vi "Post-Reanimate Hook.vi"(8 "Error In":errorcluster) -> (0 "Error Out":errorcluster)   [LabVIEW 2018, in "Tests.lvlib" / "Toolkit.lvlib" / "Integration.lvlib"]
uses:
  Integration.lvlib
  Hooks/Post-Reanimate.vi
  Support/Reanimate Target.vi
  <vilib>/addons/_JKI Toolkits/Caraya/classes/Test/Test.lvclass
  Tests.lvlib
  <vilib>/addons/_JKI Toolkits/Caraya/classes/Assert/Assert.lvclass
  src/Toolkit/Toolkit.lvlib
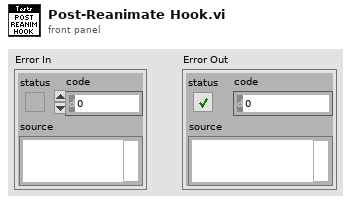
[diagram p1: front panel]
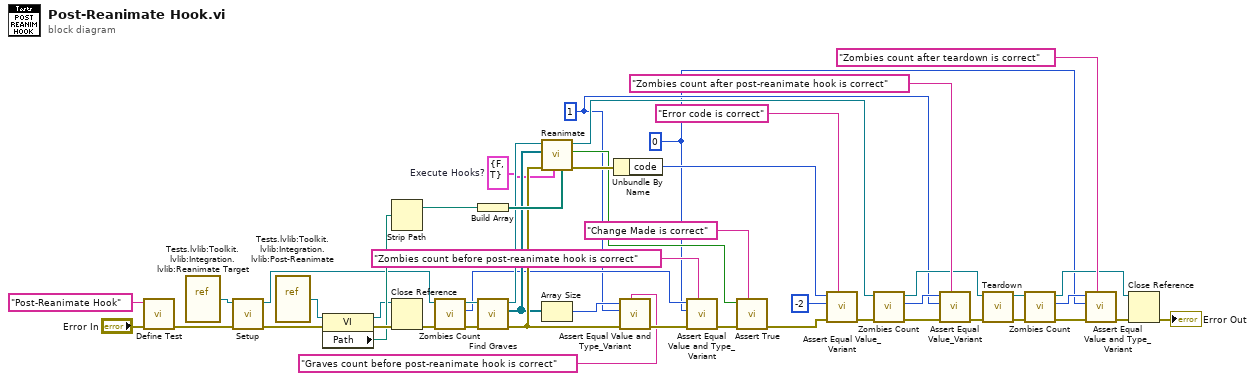
[diagram p0: block diagram]
diagram:
  w2 = 1 ("size(s)")
  w16 = cluster{"Pre":bool, "Post":bool} {"Pre"=FALSE, "Post"=TRUE}  # Execute Hooks?
  w1 = 0 ("size(s)")
  n1 = call <vilib>:"Define Test.vi"("error in (no error)"="Error In", "Label (VI Title)"="Post-Reanimate Hook") -> ("error out"=w44:errorcluster)  [unwired: 9 in]
  n2 = vi-ref "Tests.lvlib:Toolkit.lvlib:Integration.lvlib:Reanimate Target.vi"() -> (w11:refnum<vi>)
  n3 = call "Setup.vi"("Error In"=w44, "VI In"=w11) -> ("Error Out"=w36:errorcluster, "VI Out"=w28:refnum<vi>)  [unwired: 8 in]
  n4 = vi-ref "Tests.lvlib:Toolkit.lvlib:Integration.lvlib:Post-Reanimate.vi"() -> (w12:refnum<vi>)
  n5 = property class="VI"(reference=w12, error in=w36) -> (reference out=w32:refnum<vi>, error out=w35:errorcluster, "Path"=w34:path)
  n6 = Strip Path(path=w34) -> (stripped path=w33:path)  [unwired: 1 out]
  n7 = Close Reference(reference=w32, error in (no error)=w35) -> (error out=w9:errorcluster)
  n8 = call "Zombies Count.vi"("Error In"=w9, "Test Target In"=w28) -> ("Error Out"=w8:errorcluster, "Zombies Count"=w3:i32, "Test Target Out"=w10:refnum<vi>)  [unwired: 7 in]
  n9 = Build Array(w33) -> (w29:path[])
  n10 = call "Find Graves.vi"("Error In"=w8, "VI In"=w10) -> ("Error Out"=w26:errorcluster, "Graves"=w25:refnum<vi>[], "VI Out"=w27:refnum<vi>)  [unwired: 7 in]
  n11 = call "Reanimate.vi"("Hook Search Path"=w29, "Execute Hooks?"=w16, "Error In"=w26, "Graves"=w25, "VI In"=w27) -> ("Error Out"=w23:errorcluster, "Change Made?"=w14:bool, "VI Out"=w18:refnum<vi>)  [unwired: 4 in]
  n12 = Array Size(array=w25) -> (size(s)=w24:i32)
  n13 = Unbundle By Name(w23) -> ("code"=w31:i32)
  n14 = call <vilib>:"Assert Equal Value and Type_Variant.vi"("Label"="Graves count before post-reanimate hook is correct", "error in (no error)"=w26, "Y"=w2, "X"=w24) -> ("error out"=w7:errorcluster)  [unwired: 7 in]
  n15 = call <vilib>:"Assert Equal Value and Type_Variant.vi"("Label"="Zombies count before post-reanimate hook is correct", "error in (no error)"=w7, "Y"=w1, "X"=w3) -> ("error out"=w6:errorcluster)  [unwired: 7 in]
  n16 = call <vilib>:"Assert True.vi"("Label"="Change Made is correct", "error in (no error)"=w6, "True?"=w14) -> ("error out"=w15:errorcluster)  [unwired: 8 in]
  n17 = call <vilib>:"Assert Equal Value_Variant.vi"("Label"="Error code is correct", "error in (no error)"=w15, "Y"=-2 ("code"), "X"=w31) -> ("error out"=w22:errorcluster)  [unwired: 7 in]
  n18 = call "Zombies Count.vi"("Error In"=w22, "Test Target In"=w18) -> ("Error Out"=w21:errorcluster, "Zombies Count"=w20:i32, "Test Target Out"=w19:refnum<vi>)  [unwired: 7 in]
  n19 = call <vilib>:"Assert Equal Value_Variant.vi"("Label"="Zombies count after post-reanimate hook is correct", "error in (no error)"=w21, "Y"=w2, "X"=w20) -> ("error out"=w17:errorcluster)  [unwired: 7 in]
  n20 = call "Teardown.vi"("Error In"=w17, "VI In"=w19) -> ("Error Out"=w39:errorcluster, "VI Out"=w41:refnum<vi>)  [unwired: 8 in]
  n21 = call "Zombies Count.vi"("Error In"=w39, "Test Target In"=w41) -> ("Error Out"=w38:errorcluster, "Zombies Count"=w37:i32, "Test Target Out"=w40:refnum<vi>)  [unwired: 7 in]
  n22 = call <vilib>:"Assert Equal Value and Type_Variant.vi"("Label"="Zombies count after teardown is correct", "error in (no error)"=w38, "Y"=w1, "X"=w37) -> ("error out"=w43:errorcluster)  [unwired: 7 in]
  n23 = Close Reference(reference=w40, error in (no error)=w43) -> (error out=→"Error Out":errorcluster)
